vi "USRP_multi_Emitter_200MHz_16_4.vi"() -> ()   [LabVIEW 2021]
doc: "Acquires data from the Rx ports and streams the data to the host while receiving data from the host and generating the resulting waveform at the Tx ports of the NI USRP-294x/295x device. Use this VI as a template for the Simple NI-USRP Streaming sample project."
uses:
  <instrlib>/_niInstr/Register Bus/v1/FPGA/Public/Read Cmd Data.ctl
  <instrlib>/_niInstr/DSP/v1/Shared/Public/IQ Gain.ctl
  <instrlib>/_niInstr/DSP/v1/Shared/Public/IQ Impairments.ctl
  pulse_tx_vis/pdw.ctl
  pulse_tx_vis/CTL/mode_type.ctl
  <vilib>/Platform/TimedLoop/XDataNode/timing_clust.ctl
  <vilib>/Platform/TimedLoop/XDataNode/nitl_modes.ctl
  <vilib>/Platform/TimedLoop/XDataNode/wakeup.ctl
  <vilib>/rvi/Emulation/niFpgaSctlEmulationGetInTimedLoop.vi
  <vilib>/rvi/Emulation/niFpgaEmulationReportErrorSimple.vi
  <vilib>/rvi/Emulation/niFpgaGetClockAttributes.vi
  <vilib>/rvi/Emulation/niFpgaCriticalErrorInLSC.vi
  <instrlib>/_niInstr/DSP/v1/FPGA/Public/Sub VIs/Digital Gain/Digital Gain Base.vi
  <instrlib>/_niInstr/DSP/v1/FPGA/Public/Sub VIs/IQ Impairments/IQ Impairments - 1 spc.vi
  <instrlib>/_niInstr/DSP/v1/FPGA/Public/Sub VIs/Data Conversion/IQ to I16 - 1 spc - S18.1.vi
  <vilib>/rvi/eio/common/nirviEmuTemplateMethod_errors.vi
  <vilib>/rvi/interface/RandomDataEmulation/nirviRandomDataMultiElementFPGAFIFO.vi
  <instcachedir>/0/nirviRandomDataMultiElementFPGAFIFO_3E9965BA1FAD4E7B8DABA31768A09B1F.lvgen/nirviRandomDataMultiElementFPGAFIFO_3E9965BA1FAD4E7B8DABA31768A09B1F_000.vi
  <vilib>/rvi/interface/RandomDataEmulation/niFpgaRandomDataHandleErrors.vi
  <vilib>/Platform/TimedLoop/XDataNode/XDataNode.xnode
  <instrlib>/_niInstr/DSP/v1/XNodes/Public/Digital Gain/niInstr DSP v1 Digital Gain FPGA.xnode
  <instrlib>/_niInstr/DSP/v1/Shared/Public/IQ Data.ctl
  <instrlib>/_niInstr/DSP/v1/XNodes/Public/IQ Impairments/niInstr DSP v1 IQ Impairments FPGA.xnode
  <vilib>/eio/EIONode/EIONode.xnode
  <vilib>/rvi/DataTransferAndStorage/Container/XNode/niFpgaContainer.xnode
  <vilib>/rvi/interface/RandomDataEmulation/nirviRandomDataFpgaMultiElementTemplate.vi
  <vilib>/Platform/TimedLoop/XDataNode/XDNodeRunTimeDep.lvlib
  <instrlib>/_niInstr/Register Bus/v1/FPGA/niInstr Register Bus v1 FPGA.lvlib
  <instrlib>/niUsrpRio/Config/v1/FPGA/niUsrpRio Config v1 FPGA.lvlib
  <instrlib>/_niInstr/DSP/v1/Shared/niInstr DSP v1 Shared.lvlib
  <instrlib>/_niInstr/DSP/v1/FPGA/niInstr DSP v1 FPGA.lvlib
panel:
  out "debug mode":T3 {"Cluster"."frequency shift" format="%#_12f"}
  out "pulse TX status":T4
  in  "IQ_run":bool=TRUE
  in  "LED/RF 1/TX1 RX1":enum8{"Off", "Green", "Red", "Amber"}(ring)
  in  "LED/RF 0/TX1 RX1":enum8{"Off", "Green", "Red", "Amber"}(ring)
  in  "tx.impairments.0":T5={"inline gain I"=0.9999923706054688, "inline gain Q"=0.9999923706054688, "cross gain I"=0.0, "cross gain Q"=0.0, "pre-gain offset I"=0.0, "pre-gain offset Q"=0.0, "post-gain offset I"=0.0, "post-gain offset Q"=0.0}
  in  "tx.gain.0":T6={"gain I"=1.0, "gain Q"=1.0}
  in  "reset system clock":bool
  in  "RF 1/Tx/Enable":bool
  in  "RF 1/Rx/Enable":bool
  in  "RF 0/Tx/Enable":bool
  in  "RF 0/Rx/Enable":bool
  in  "reg.host read.go rcvd 0":bool
  out "reg.notify host.go 0":bool
  in  "reg.notify host.go rcvd 0":bool
  out "reg.host read.data 0":T7
  in  "reg.reset 0":bool
  # "USRP RIO pulse Streaming FPGA"
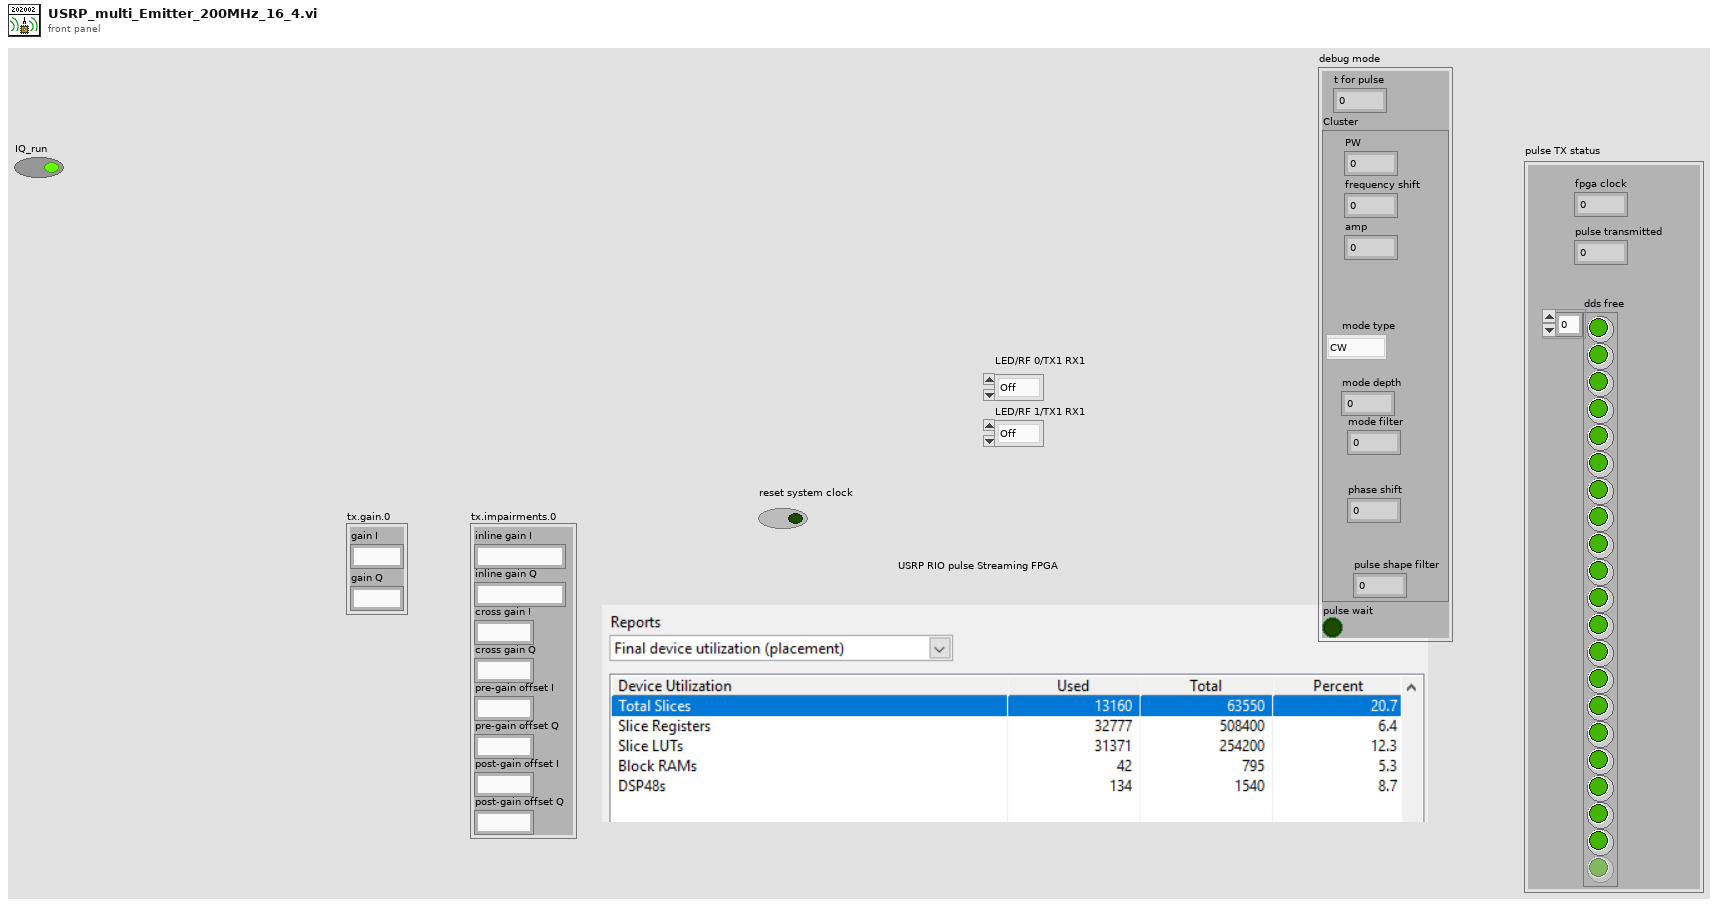
[diagram p1: front panel]
types:
  T1 = typedef "pdw.ctl" = cluster{"PW":u32, "frequency shift":fxp<+/-,48,0>, "amp":fxp<+/-,18,1>, "mode type":T2, "mode depth":u32, "mode filter":u8, "phase shift":fxp<+/-,16,1>, "pulse shape filter":u8}
  T2 = typedef "mode_type.ctl" = enum8{"CW", "from memory 1", "NC - cw", "LFM", "BPSK", "QPSK"}
  T3 = cluster{"t for pulse":u64, "Cluster":T1, "pulse wait":bool}
  T4 = cluster{"fpga clock":u64, "pulse transmitted":u32, "dds free":bool[]}
  T5 = typedef "niInstr DSP v1 Shared.lvlib/IQ Impairments.ctl" = cluster{"inline gain I":fxp<+/-,18,1>, "inline gain Q":fxp<+/-,18,1>, "cross gain I":fxp<+/-,18,1>, "cross gain Q":fxp<+/-,18,1>, "pre-gain offset I":fxp<+/-,18,1>, "pre-gain offset Q":fxp<+/-,18,1>, "post-gain offset I":fxp<+/-,18,1>, "post-gain offset Q":fxp<+/-,18,1>}
  T6 = typedef "niInstr DSP v1 Shared.lvlib/IQ Gain.ctl" = cluster{"gain I":fxp<+/-,24,3>, "gain Q":fxp<+/-,24,3>}
  T7 = typedef "niInstr Register Bus v1 FPGA.lvlib/Read Cmd Data.ctl" = cluster{"go":bool, "data":u32}
  T8 = typedef "XDNodeRunTimeDep.lvlib/timing_clust.ctl" = cluster{"Expected End [f-1]":u64, "Actual End [f-1]":u64, "Finished Late? [f-1]":bool, "Expected End [i-1]":u64, "Actual End [i-1]":u64, "Finished Late? [i-1]":bool, "Expected Start [i]":u64, "Actual Start [i]":u64, "Expected Start [f]":u64, "Actual Start [f]":u64, "Source Name":string, "Structure Name":string, "Period":i64, "Deadline":i64, "Offset":i64, "Start":i64, "Priority":i32, "Timeout":i32, "Mode":T9, "Wakeup Reason":T10, "Error":errorcluster, "Source Type":string, "Secondary Source Type":string, "Global End Time":u64, "Global Start Time":u64, "Frame Duration":u64, "Iteration Duration":u64, "Assigned CPU":i32, "I/O Scan Engine Mode":u32}
  T9 = typedef "XDNodeRunTimeDep.lvlib/nitl_modes.ctl" = enum32{"No Change", "Process missed periods, maintain original phase", "Discard missed periods, maintain original phase", "Process missed periods, ignore original phase", "Discard missed periods, ignore original phase"}
  T10 = typedef "XDNodeRunTimeDep.lvlib/wakeup.ctl" = enum32{"Normal", "Aborted", "Asynchronous wakeup", "Timing source error", "Timed loop error", "Timeout"}
  T11 = cluster{"Memory In":refnum<k21>, "Memory In 2":refnum<k21>, "Memory In 3":refnum<k21>, "Memory In 6":refnum<k21>}
  T12 = cluster{"clock x2":refnum<k21>, "Memory In":refnum<k21>, "Memory In 2":refnum<k21>, "Memory In 3":refnum<k21>, "Memory In 4":refnum<k21>}
  T13 = typedef "niInstr DSP v1 Shared.lvlib/IQ Data.ctl" = cluster{"I":fxp<+/-,18,1>, "Q":fxp<+/-,18,1>, "overflow":bool}
  T14 = cluster{"DAC FIFO Reset":refnum<k21>, "RF 0 Rx Swap IQ":refnum<k21>, "RF 0 Rx Negate I":refnum<k21>, "RF 0 Rx Negate Q":refnum<k21>, "RF 0 Rx Data Valid":refnum<k21>, "RF 0 Rx Data Ever Invalid":refnum<k21>, "clear RF 0 Rx Data Ever Invalid":refnum<k21>, "RF 0 Tx Swap IQ":refnum<k21>, "RF 0 Tx Negate I":refnum<k21>, "RF 0 Tx Negate Q":refnum<k21>, "RF 1 Rx Swap IQ":refnum<k21>, "RF 1 Rx Negate I":refnum<k21>, "RF 1 Rx Negate Q":refnum<k21>, "RF 1 Rx Data Valid":refnum<k21>, "RF 1 Rx Data Ever Invalid":refnum<k21>, "clear RF 1 Rx Data Ever Invalid":refnum<k21>, "RF 1 Tx Swap IQ":refnum<k21>, "RF 1 Tx Negate I":refnum<k21>, "RF 1 Tx Negate Q":refnum<k21>}
  T15 = typedef "niUsrpRio Synchronization v1 FPGA.lvlib/Resources.ctl" = cluster{"master":refnum<k21>, "meas.enable":refnum<k21>, "meas.ready":refnum<k21>, "meas.reset":refnum<k21>, "meas.arm":refnum<k21>, "meas.valid":refnum<k21>, "meas.value":refnum<k21>, "meas.oversample factor":refnum<k21>, "cptr":refnum<k21>, "cptr.adjust":refnum<k21>, "cptr.period":refnum<k21>}
  T16 = typedef "niUsrpRio Time v1 FPGA.lvlib/Time Resources.ctl" = cluster{"reset":refnum<k21>, "time":refnum<k21>, "time.previous cptr":refnum<k21>, "new time":refnum<k21>, "new time.when":refnum<k21>, "new time.set":refnum<k21>, "which edge of ref":refnum<k21>, "pps source":refnum<k21>, "internal pps period":refnum<k21>}
  T17 = typedef "niUsrpRio Time v1 FPGA.lvlib/Future Event Resources.ctl" = cluster{"reset":refnum<k21>, "future event.time":refnum<k21>, "future event.ready":refnum<k21>, "future event.set":refnum<k21>, "future event.clear":refnum<k21>, "future event.set in past":refnum<k21>}
  T18 = cluster{"time.resources":T16, "future event.resources":T17, "future event.resources":T17}
  T19 = typedef "niInstr Register Bus v1 FPGA.lvlib/Register Instruction.ctl" = cluster{"subsystem":u8, "address":u16, "data":u32, "valid":bool, "read":bool}
  T20 = typedef "niInstr Register Bus v1 FPGA.lvlib/Read Completion.ctl" = cluster{"data":u32, "valid":bool}
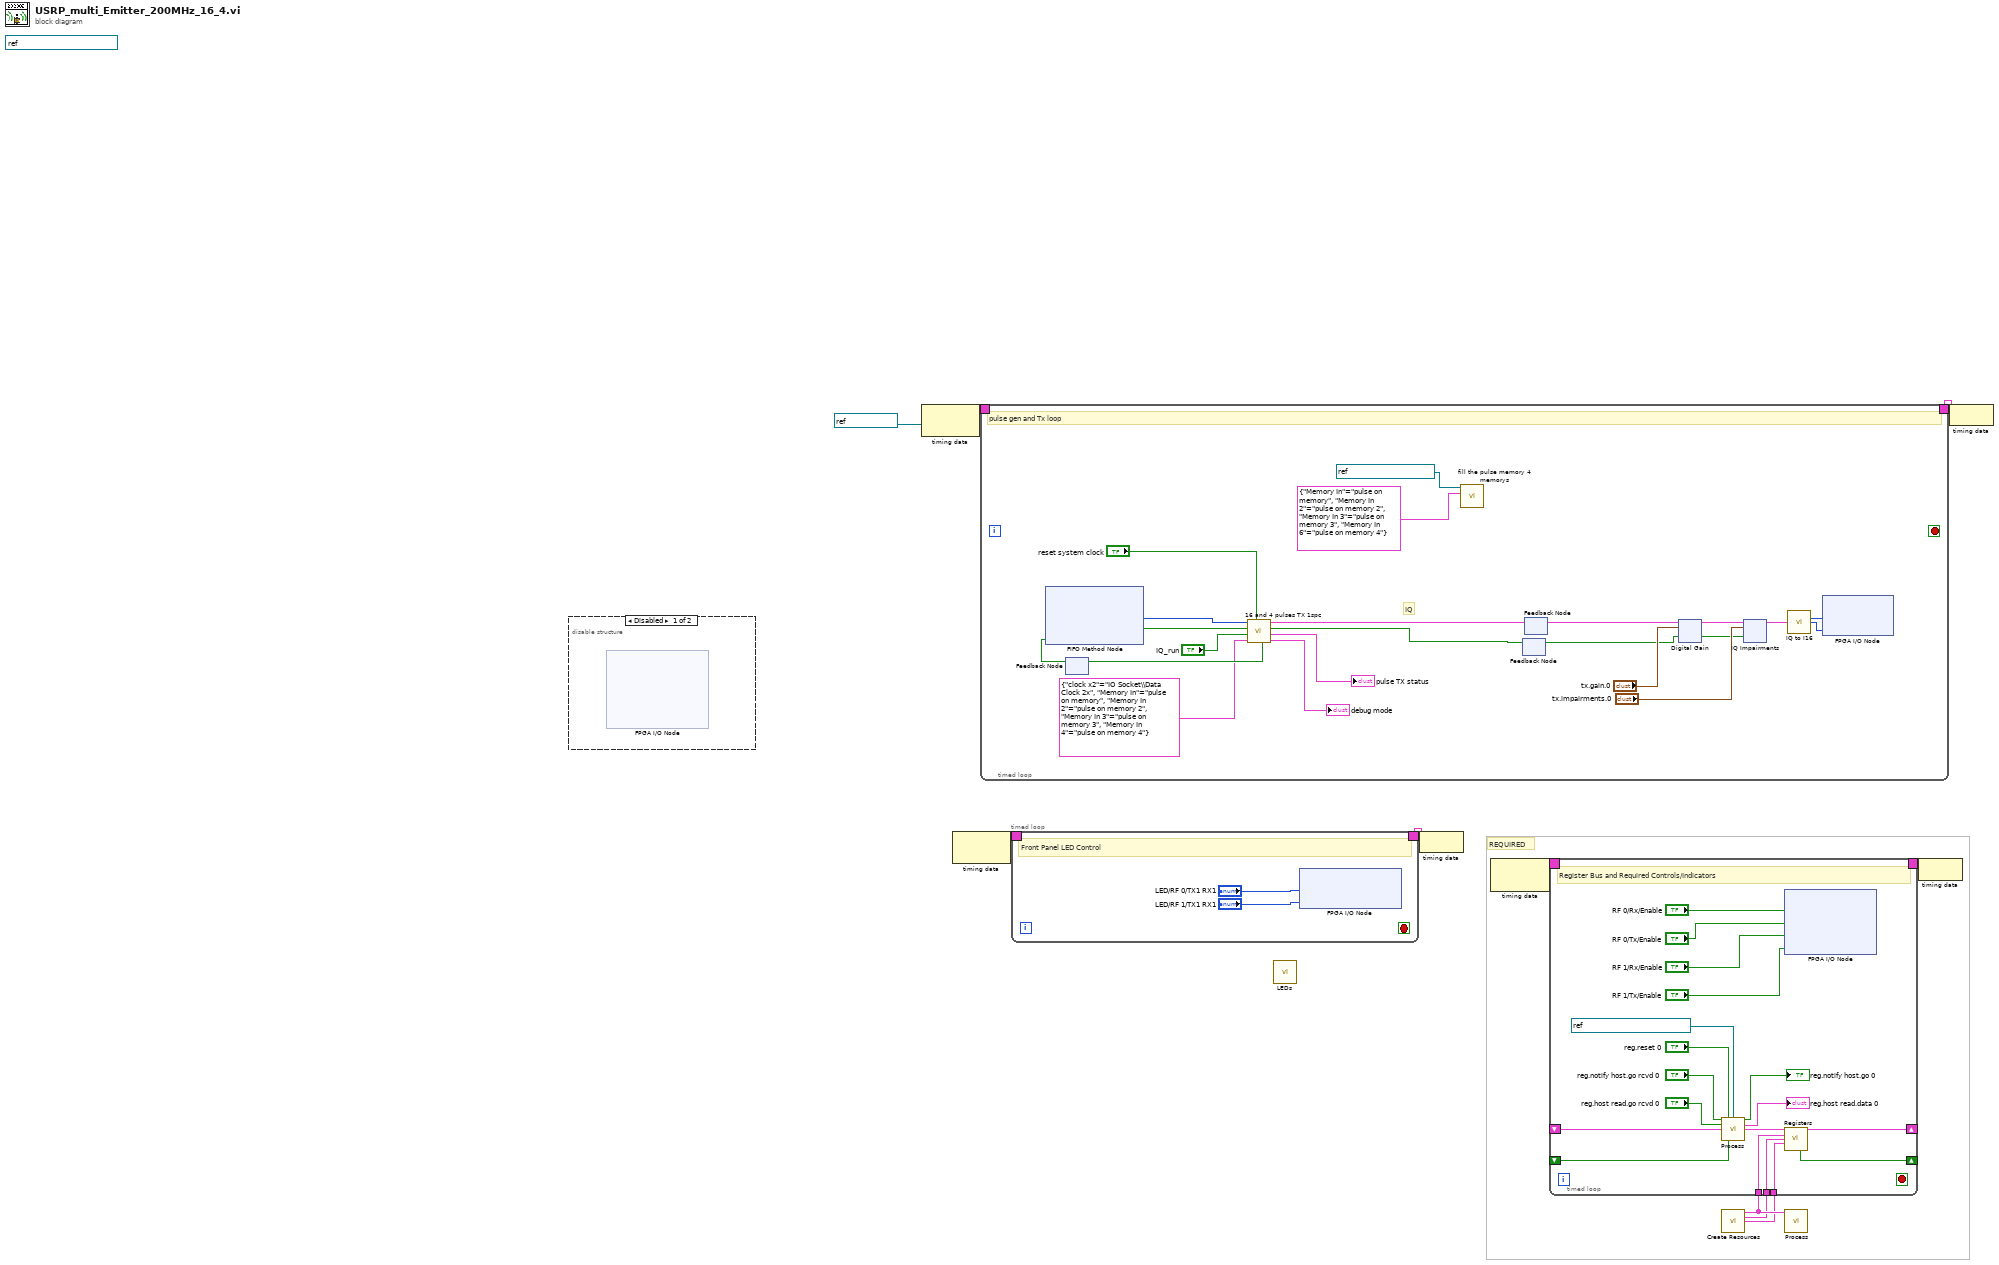
[diagram p0: block diagram]
diagram:
  (unwired) refnum<k21> "40 MHz Onboard Clock" ("Source Name")
  # "REQUIRED"
  n1 = disable-structure shown="Disabled" {
    frame Disabled {
      n2 = xnode "FPGA I/O Node"() -> ()  [unwired: 10 in, 5 out]
    }
    frame Enabled {
    }
  }
  n3 = node-c288(refnum<k21> "Data Clock" ("Source Name")) -> (w3:T8)
  n4 = node-c288() -> (w5:T8)  [unwired: 1 in]
  n5 = timed-loop {
    timing: w3 -> [_]
    timing-out: [_] -> w2
    stop <- _ stop-if-true
    # "IQ"
    # "pulse gen and Tx loop"
    n6 = feedback #1() -> (w28:bool)  [unwired: 1 in]
    n7 = xnode ("FIFO Method Node")("Ready for Output"=w28) -> ("Element"=w31:u64[], "Output Valid"=w32:bool)  [unwired: 1 in, 1 out]
    n8 = call "16 and 4 pulses TX 1spc.vi"("reset system clock"="reset system clock", "referenses"=T12 {"clock x2"="IO Socket\\Data Clock 2x", "Memory In"="pulse on memory", "Memory In 2"="pulse on memory 2", "Memory In 3"="pulse on memory 3", "Memory In 4"="pulse on memory 4"}, "IQ_run"="IQ_run", "PDW input Valid"=w32, "array PDW"=w31) -> ("debug mode"=→"debug mode":T3, "pulse TX status"=→"pulse TX status":T4, "output valid"=w17:bool, "IQ out"=w20:T13, "ready for input"=w29:bool)  [unwired: 2 in]
    n9 = feedback-in #1(w29) -> ()
    n10 = call "fill the pulse memory 4 memorys.vi"("memory units"=T11 {"Memory In"="pulse on memory", "Memory In 2"="pulse on memory 2", "Memory In 3"="pulse on memory 3", "Memory In 6"="pulse on memory 4"}, "FIFO In"=refnum<k21> "fifo pulse from host") -> ()  [unwired: 10 in]
    n11 = feedback #2() -> (w16:bool)  [unwired: 1 in]
    n12 = feedback-in #2(w17) -> ()
    n13 = feedback #3() -> (w19:T13)  [unwired: 1 in]
    n14 = feedback-in #3(w20) -> ()
    n15 = xnode "Digital Gain"("data in"=w19, "gain"="tx.gain.0", "input valid"=w16) -> ("data out"=w24:T13, "output valid"=w23:bool)  [unwired: 2 in, 1 out]
    n16 = xnode "IQ Impairments"("data in"=w24, "impairments"="tx.impairments.0", "input valid"=w23) -> ("data out"=w25:T13)  [unwired: 2 in, 2 out]
    n17 = call-poly <instrlib>:"IQ to I16.vi"("IQ"=w25) -> ("I"=w21:i16, "Q"=w22:i16)  [unwired: 12 in, 1 out]
    n18 = xnode "FPGA I/O Node"("RF 0/Tx/I"=w21, "RF 0/Tx/Q"=w22) -> ()  [unwired: 2 in, 2 out]
  }
  n19 = timed-loop {
    timing: w5 -> [_]
    timing-out: [_] -> w4
    stop <- _ stop-if-true
    # "Front Panel LED Control"
    n20 = xnode "FPGA I/O Node"("LED/RF 0/TX1 RX1"="LED/RF 0/TX1 RX1", "LED/RF 1/TX1 RX1"="LED/RF 1/TX1 RX1") -> ()  [unwired: 2 in, 2 out]
  }
  n21 = call <instrlib>:"LEDs.vi"() -> ()  [unwired: 1 in]
  n22 = node-c288(w4) -> ()
  n23 = node-c288() -> (w10:T8)  [unwired: 1 in]
  n24 = call <instrlib>:"Create Resources.vi"() -> ("config.resources"=w8:T14, "sync.resources"=w7:T15, "time.resources"=w6:T18)  [unwired: 13 in]
  n25 = timed-loop "Register Bus and Required Controls/Indicators" {
    timing: w10 -> [_]
    timing-out: [_] -> w9
    shift-right: [w70] -> _
    shift-left: _ -> [w69]
    shift-right: [w64] -> _
    shift-left: _ -> [w68]
    tunnel: w8 -> [w62]
    tunnel: w7 -> [w61]
    tunnel: w6 -> [w60]
    stop <- _ stop-if-true
    # "Register Bus and Required Controls/Indicators"
    n26 = call <instrlib>:"Process.vi"("reg.notify host.go rcvd"="reg.notify host.go rcvd 0", "reg.reset"="reg.reset 0", "reg.host instruction fifo"=refnum<k21> "reg.host instruction fifo 0", "reg.host read.go rcvd"="reg.host read.go rcvd 0", "read completion"=w69, "ready for output"=w68) -> ("reg.notify host.go"=→"reg.notify host.go 0":bool, "reg.host read.data"=→"reg.host read.data 0":T7, "register instruction"=w63:T19)  [unwired: 7 in]
    n27 = xnode ("FPGA I/O Node")("RF 0/Rx/Enable"="RF 0/Rx/Enable", "RF 0/Tx/Enable"="RF 0/Tx/Enable", "RF 1/Rx/Enable"="RF 1/Rx/Enable", "RF 1/Tx/Enable"="RF 1/Tx/Enable") -> ()  [unwired: 4 in, 4 out]
    n28 = call <instrlib>:"Registers.vi"("register instruction"=w63, "config.resources"=w62, "sync.resources"=w61, "time.resources"=w60) -> ("read completion out"=w70:T20, "ready for input"=w64:bool)  [unwired: 10 in]
  }
  n29 = call <instrlib>:"Process.vi"("resources"=w8) -> ()  [unwired: 15 in]
  n30 = node-c288(w9) -> ()
  n31 = node-c288(w2) -> ()
